vi "Swerve Out of loop.vi"(0 "x":dbl(slide)=-0.03937007874015748 scale=-1.0..1.0, 1 "Recalc offsets":bool, 2 "Recalc distance":bool, 5 "Rot. Point X":dbl, 7 "y":dbl(slide)=-0.07086614173228346 scale=-1.0..1.0, 9 "Rot. Point Y":dbl, 11 "z":dbl(knob)=-0.015748031496062992 scale=-1.0..1.0, 12 "Robot Centric":bool=TRUE, 13 "Auto Controls":bool) -> ()   [LabVIEW 2016]
uses:
  <vilib>/Rock Robotics/WPI/ThirdParty/CanMotor/TalonSRX/WPI_CANTalonSRX_APIControlMode.ctl
  <vilib>/Rock Robotics/WPI/ThirdParty/CanMotor/TalonSRX/WPI_CANTalonSRX_APIFeedbackSelect.ctl
  <vilib>/Rock Robotics/WPI/ThirdParty/CanMotor/TalonSRX/WPI_CANTalonSRX_StatusFrame.ctl
  <vilib>/Rock Robotics/Network Tables/NT Read Number.vi
  <vilib>/Rock Robotics/Network Tables/NT Read Numeric Array.vi
panel:
  in  "Default Offsets":dbl[](array[numeric])=[0.0987354, 0.084183, 0.097507, -0.49821]
  in  "negate feedback sensor":bool
  in  "Deadband":dbl=0.04 format="%#_13g"
  in  "Debug?":bool
  in  "Motor":bool[](array[boolean])=[FALSE, FALSE, FALSE, FALSE]
  in  "PIDF":cluster{"P":dbl, "I":dbl, "D":dbl, "F":dbl}={"P"=2.0, "I"=0.0, "D"=0.0, "F"=0.0}
  in  "Robot Width":dbl=26.0
  in  "Robot Length":dbl=22.125
  # "SWERVE DRIVE\nVersion 4.0\nCory Lynch\nChris Garuti\nGavin Popkin\nApple Pi Robotics\nTeam 2067"
  # "FL"
  # "FR"
  # "BL"
  # "BR"
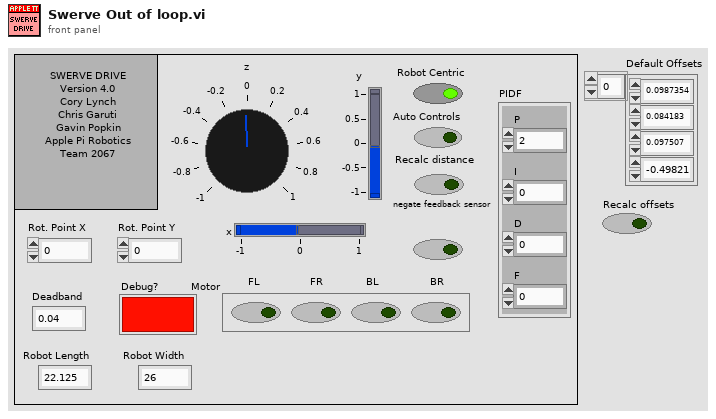
[diagram p1: front panel]
types:
  T1 = typedef "WPI_MotorControlDeviceRef.ctl" = cluster{"DeviceStatus":errorcluster, "Type":T2, "PWM":cluster{"PWM Channel":T3, "DeadBand":T4}, "CAN":cluster{"Device Number":u8, "SetOutput VI Ref":variant, "GetOutput VI Ref":variant, "Enable VI Ref":variant, "Disable VI Ref":variant, "Data":variant}, "Invert":bool}
  T2 = typedef "WPI_MotorControlType.ctl" = enum16{"PWM", "CAN"}
  T3 = typedef "FPGA_DIOPWMChannel.ctl" = enum8{"PWM 0", "PWM 1", "PWM 2", "PWM 3", "PWM 4", "PWM 5", "PWM 6", "PWM 7", "PWM 8", "PWM 9", "PWM MXP 0", "PWM MXP 1", "PWM MXP 2", "PWM MXP 3", "PWM MXP 4", "PWM MXP 5", "PWM MXP 6", "PWM MXP 7", "PWM MXP 8", "PWM MXP 9", "Invalid"}
  T4 = typedef "WPI_PWMDeadband.ctl" = cluster{"Name":string, "maxPositivePwm":i32, "minPositivePwm":i32, "centerPwm":i32, "maxNegativePwm":i32, "minNegativePwm":i32, "angularRange":u16}
  T5 = typedef "WPI_CANTalonSRX_StatusFrame.ctl" = enum16{"General Status Frame", "Feedback Status Frame", "Quadrature Status Frame", "Analog Temp Vbat Status Frame", "Pulse Width Status Frame"}
  T6 = typedef "WPI_CANTalonSRX_APIFeedbackSelect.ctl" = enum16{"Digital Quadrature Encoder", "Analog Potentiometer", "Analog Encoder", "Count on Quad-A (Rising-Edge)", "Count on Quad-A (Falling-Edge)", "CTR Magnetic Enc (Absolute)", "CTR Magnetic Enc (Relative)", "Pulse Width"}
  T7 = typedef "WPI_CANTalonSRX_GlobalStatus.ctl" = cluster{"Applied Throttle":dbl, "Module Enabled":bool, "CAN Error":errorcluster, "Closed Loop Error":dbl, "Forward Limit Switch Closed":bool, "Reverse Limit Switch Closed":bool, "Sensor Position":dbl, "Sensor Velocity":dbl, "Current":dbl, "Sticky Fault - Over Temp":bool, "Sticky Fault - Under Voltage":bool, "Sticky Fault - Forward Limit":bool, "Sticky Fault - Reverse Limit":bool, "Sticky Fault - Forward Soft Limit":bool, "Sticky Fault - Reverse Soft Limit":bool, "Brake is Enabled":bool, "Encoder Position":dbl, "Encoder Velocity":dbl, "Encoder Index Count":dbl, "Encoder A Pin State":bool, "Encoder B Pin State":bool, "Encoder Index Pin State":bool, "Analog In":dbl, "Analog In Velocity":dbl, "Temperature (C)":dbl, "Battery Voltage":dbl, "Control 5 Is Supported":bool, "Current Profile Slot Select":dbl, "Pos Div 8":bool, "Vel Div 4":bool, "Pulse Width Position":i32, "Pulse Width Velocity":i32, "Pulse Width Rise To Rise (us)":i32, "Pulse Width Rise To Fall (us)":i32, "Mot Prof Active Is Under Run":bool, "Mot Prof Active Has Under Run":bool, "Mot Prof Active Is Last":bool, "Mot Prof Active Velocity Only":bool, "Mot Prof Active Is Valid":bool, "Mot Prof Buffer Is Full":bool, "Mot Prof Active Profile Slot Select":i32, "Mot Prof NextID":i32, "Mot Prof Count":i32, "Mot Prof Active Velocity":dbl, "Mot Prof Active Position":dbl, "Mot Prof Output Enable":i32, "UsageFrame":u32, "Motion Magic Active Trajectory":cluster{"Velocity":dbl, "Position":dbl}}
  T8 = typedef "WPI_CANTalonSRX_APIControlMode.ctl" = enum8{"Percent VBus", "Speed", "Position", "Slave", "Unchanged / Invalid", "Voltage Compensation", "Current", "Motion Profile", "Motion Magic"}
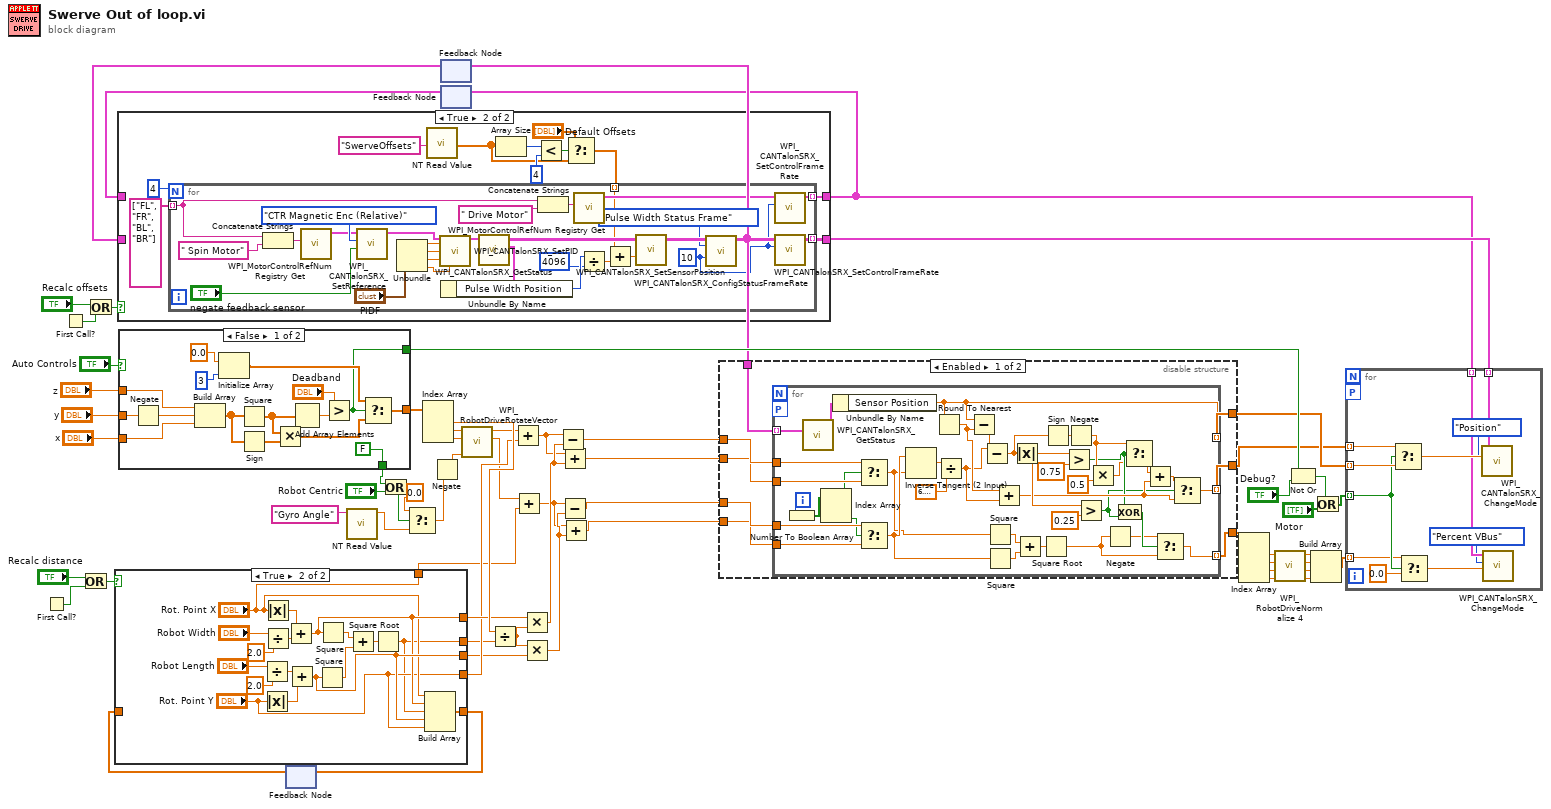
[diagram p0: block diagram]
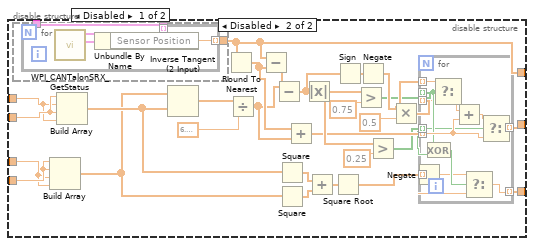
[diagram p2: hidden frame]
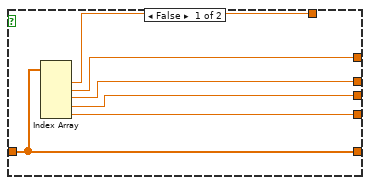
[diagram p5: hidden frame]
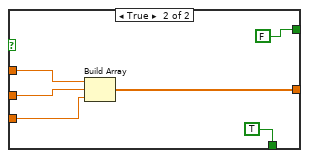
[diagram p6: hidden frame]
diagram:
  n1 = First Call?() -> (First Call?: T/F=w38:bool)
  n2 = First Call?() -> (First Call?: T/F=w12:bool)
  n3 = Or(x="Recalc distance", y=w38) -> (x .or. y?=w36:bool)
  n4 = Or(x="Recalc offsets", y=w12) -> (x .or. y?=w39:bool)
  n5 = case shown="False" "Auto Controls" {
    tunnel: [w71 w83] -> w61
    tunnel: [w67 FALSE] -> w51
    tunnel: "z" -> [w65 w81]
    tunnel: "y" -> [w64 w80]
    tunnel: "x" -> [w63 w79]
    tunnel: [FALSE TRUE] -> w3
    frame False {
      n6 = Negate(x=w64) -> (-x=w66:dbl)
      n7 = Build Array(w65, w66, w63) -> (w75:dbl[])
      n8 = Initialize Array(0.0 ("element"), 3 ("dimension size")) -> (w77:dbl[])
      n9 = Square(x=w75) -> (x^2=w73:dbl[])
      n10 = Sign(1:w75) -> (0:w74:dbl[])
      n11 = Multiply(x=w73, y=w74) -> (x*y=w72:dbl[])
      n12 = Add Array Elements(numeric array=w73) -> (sum=w69:dbl)
      n13 = Greater?(x="Deadband", y=w69) -> (0:w67:bool)
      n14 = Select(t=w77, s=w67, f=w72) -> (s? t:f=w71:dbl[])
    }
    frame True {
      n15 = Build Array(w81, w80, w79) -> (w83:dbl[])
    }
  }
  n16 = feedback #1() -> (w20:dbl[])  [unwired: 1 in]
  n17 = case shown="True" w36 {
    tunnel: [w88 w94] -> w58
    tunnel: [w85 "Rot. Point Y"] -> w57
    tunnel: [w89 "Rot. Point X"] -> w30
    tunnel: [w87 w90] -> w55
    tunnel: [w86 w95] -> w56
    tunnel: [w84 w91] -> w19
    tunnel: w20 -> [w84 _]
    frame False {
      n18 = Index Array(array=w84) -> (element #1=w89:dbl, element #2=w88:dbl, element #3=w87:dbl, element #4=w86:dbl, element #5=w85:dbl)  [unwired: 5 in]
    }
    frame True {
      n19 = Divide(x="Robot Length", y=2.0) -> (x/y=w98:dbl)
      n20 = Absolute Value(x="Rot. Point Y") -> (abs(x)=w97:dbl)
      n21 = Absolute Value(x="Rot. Point X") -> (abs(x)=w96:dbl)
      n22 = Divide(x="Robot Width", y=2.0) -> (x/y=w99:dbl)
      n23 = Add(x=w96, y=w99) -> (x+y=w94:dbl)
      n24 = Add(x=w98, y=w97) -> (x+y=w95:dbl)
      n25 = Square(x=w95) -> (x^2=w101:dbl)
      n26 = Square(x=w94) -> (x^2=w104:dbl)
      n27 = Add(x=w104, y=w101) -> (x+y=w105:dbl)
      n28 = Square Root(x=w105) -> (sqrt(x)=w90:dbl)
      n29 = Build Array("Rot. Point X", w94, w90, w95, "Rot. Point Y") -> (w91:dbl[])
    }
  }
  n30 = feedback-in #1(w19) -> ()
  n31 = call-poly <vilib>:"NT Read Value.vi"("Name"="Gyro Angle") -> ("Numeric"=w1:dbl)  [unwired: 9 in, 1 out]
  n32 = Or(x=w3, y="Robot Centric") -> (x .or. y?=w4:bool)
  n33 = Select(t=0.0, s=w4, f=w1) -> (s? t:f=w49:dbl)
  n34 = Index Array(array=w61) -> (element #1=w60:dbl, element #2=w48:dbl, element #3=w47:dbl)  [unwired: 3 in]
  n35 = Negate(x=w49) -> (-x=w11:dbl)
  n36 = feedback #2() -> (w16:T1[])  [unwired: 1 in]
  n37 = feedback #3() -> (w18:T1[])  [unwired: 1 in]
  n38 = case shown="True" w39 {
    tunnel: [w107 w119] -> w17
    tunnel: [w108 w118] -> w15
    tunnel: w18 -> [w108 _]
    tunnel: w16 -> [w107 _]
    frame False {
    }
    frame True {
      n39 = call-poly <vilib>:"NT Read Value.vi"("Name"="SwerveOffsets") -> ("Numeric Array"=w110:dbl[])  [unwired: 9 in, 1 out]
      n40 = Array Size(array=w110) -> (size(s)=w115:i32)
      n41 = Less?(x=w115, y=4) -> (x < y?=w113:bool)
      n42 = Select(t="Default Offsets", s=w113, f=w110) -> (s? t:f=w111:dbl[])
      n43 = for {
        N: 4 -> [_]
        tunnel: string[] ["FL", "FR", "BL", "BR"] -> [w142] mode=indexing
        tunnel: [w121] -> w118 mode=indexing
        tunnel: [w122] -> w119 mode=indexing
        tunnel: w111 -> [w125] mode=indexing
        w120 = u32 10 ("Frame Rate Ms")
        n44 = Concatenate Strings(w142, " Spin Motor" ("refnum name")) -> (w141:string)
        n45 = call <vilib>:"WPI_MotorControlRefNum Registry Get.vi"("refnum name"=w141) -> ("MotorControlDevRef"=w143:T1)  [unwired: 9 in, 1 out]
        n46 = call <vilib>:"WPI_CANTalonSRX_SetReference.vi"("Reverse Feedback Sensor"="negate feedback sensor", "Feedback Reference"=WPI_CANTalonSRX_APIFeedbackSelect."CTR Magnetic Enc (Relative)", "CAN Talon SRX Ref"=w143) -> ("CAN Talon SRX Ref"=w137:T1)  [unwired: 7 in, 1 out]
        n47 = Unbundle("PIDF") -> ("P"=w144:dbl, "I"=w146:dbl, "D"=w145:dbl, "F"=w135:dbl)
        n48 = call <vilib>:"WPI_CANTalonSRX_SetPID.vi"("CAN Talon SRX Ref"=w137, "P"=w144, "I"=w146, "D"=w145, "F"=w135) -> ("CAN Talon SRX Ref"=w133:T1)  [unwired: 9 in, 1 out]
        n49 = call <vilib>:"WPI_CANTalonSRX_GetStatus.vi"("CAN Talon SRX Ref"=w133) -> ("Talon SRX Status"=w130:T7, "CAN Talon SRX Ref"=w132:T1)  [unwired: 8 in, 1 out]
        n50 = Unbundle By Name(w130) -> ("Pulse Width Position"=w128:i32)
        n51 = Concatenate Strings(w142, " Drive Motor") -> (w140:string)
        n52 = call <vilib>:"WPI_MotorControlRefNum Registry Get.vi"("refnum name"=w140) -> ("MotorControlDevRef"=w139:T1)  [unwired: 9 in, 1 out]
        n53 = Divide(x=w128, y=4096) -> (x/y=w129:dbl)
        n54 = Add(x=w125, y=w129) -> (x+y=w126:dbl)
        n55 = call <vilib>:"WPI_CANTalonSRX_SetSensorPosition.vi"("New Sensor Position"=w126, "CAN Talon SRX Ref"=w132) -> ("CAN Talon SRX Ref"=w131:T1)  [unwired: 8 in, 1 out]
        n56 = call <vilib>:"WPI_CANTalonSRX_ConfigStatusFrameRate.vi"("CAN Talon SRX Ref"=w131, "Talon SRX Status Frame"=WPI_CANTalonSRX_StatusFrame."Pulse Width Status Frame", "Frame Rate Ms"=w120) -> ("CAN Talon SRX Ref"=w124:T1)  [unwired: 12 in]
        n57 = call <vilib>:"WPI_CANTalonSRX_SetControlFrameRate.vi"("Control Frame Rate (ms)"=w120, "CAN Talon SRX Ref"=w139) -> ("CAN Talon SRX Ref"=w121:T1)  [unwired: 8 in, 1 out]
        n58 = call <vilib>:"WPI_CANTalonSRX_SetControlFrameRate.vi"("Control Frame Rate (ms)"=w120, "CAN Talon SRX Ref"=w124) -> ("CAN Talon SRX Ref"=w122:T1)  [unwired: 8 in, 1 out]
      }
    }
  }
  n59 = feedback-in #2(w17) -> ()
  n60 = feedback-in #3(w15) -> ()
  n61 = call <vilib>:"WPI_RobotDriveRotateVector.vi"("Angle"=w11, "X"=w47, "Y"=w48) -> ("X'"=w45:dbl, "Y'"=w46:dbl)  [unwired: 7 out]
  n62 = Divide(x=w60, y=w55) -> (x/y=w59:dbl)
  n63 = Add(x=w46, y=w57) -> (x+y=w31:dbl)
  n64 = Add(x=w45, y=w30) -> (x+y=w32:dbl)
  n65 = Multiply(x=w58, y=w59) -> (x*y=w34:dbl)
  n66 = Multiply(x=w59, y=w56) -> (x*y=w33:dbl)
  n67 = Subtract(x=w31, y=w34) -> (x-y=w10:dbl)
  n68 = Add(x=w31, y=w34) -> (x+y=w9:dbl)
  n69 = Subtract(x=w32, y=w33) -> (x-y=w8:dbl)
  n70 = Add(x=w32, y=w33) -> (x+y=w7:dbl)
  n71 = disable-structure shown="Enabled" {
    disable-tunnel: [w156 w197] -> w35
    disable-tunnel: [w155 w198] -> w29
    disable-tunnel: [w154 w200] -> w24
    disable-tunnel: w17 -> [w153 w199]
    disable-tunnel: w10 -> [w152 w205]
    disable-tunnel: w9 -> [w151 w206]
    disable-tunnel: w8 -> [w150 w202]
    disable-tunnel: w7 -> [w149 w203]
    frame Enabled {
      n72 = for {
        tunnel: [w191] -> w155 mode=indexing
        tunnel: [w168] -> w154 mode=indexing
        tunnel: w153 -> [w188] mode=indexing
        tunnel: [w175] -> w156 mode=indexing
        tunnel: w152 -> [w182]
        tunnel: w151 -> [w183]
        tunnel: w150 -> [w185]
        tunnel: w149 -> [w184]
        workers-P: _ -> [_]
        i -> [w187]
        n73 = Number To Boolean Array(number=w187) -> (Boolean array=w186:bool[])
        n74 = call <vilib>:"WPI_CANTalonSRX_GetStatus.vi"("CAN Talon SRX Ref"=w188) -> ("Talon SRX Status"=w157:T7)  [unwired: 8 in, 2 out]
        n75 = Index Array(array=w186) -> (element #1=w159:bool, element #2=w158:bool)  [unwired: 2 in]
        n76 = Unbundle By Name(w157) -> ("Sensor Position"=w175:dbl)
        n77 = Select(t=w182, s=w159, f=w183) -> (s? t:f=w180:dbl)
        n78 = Select(t=w185, s=w158, f=w184) -> (s? t:f=w181:dbl)
        n79 = Inverse Tangent (2 Input)(1:w180, 2:w181) -> (0:w189:dbl)
        n80 = Round To Nearest(number=w175) -> (nearest integer value=w173:dbl)
        n81 = Divide(x=w189, y=6.283185307179586) -> (x/y=w172:dbl)
        n82 = Subtract(x=w175, y=w173) -> (x-y=w179:dbl)
        n83 = Subtract(x=w172, y=w179) -> (x-y=w174:dbl)
        n84 = Square(x=w180) -> (x^2=w194:dbl)
        n85 = Square(x=w181) -> (x^2=w195:dbl)
        n86 = Add(x=w173, y=w172) -> (x+y=w167:dbl)
        n87 = Absolute Value(x=w174) -> (abs(x)=w177:dbl)
        n88 = Add(x=w194, y=w195) -> (x+y=w193:dbl)
        n89 = Square Root(x=w193) -> (sqrt(x)=w192:dbl)
        n90 = Sign(1:w174) -> (0:w170:dbl)
        n91 = Greater?(x=w177, y=0.75) -> (0:w165:bool)
        n92 = Negate(x=w170) -> (-x=w166:dbl)
        n93 = Greater?(x=w177, y=0.25) -> (0:w160:bool)
        n94 = Multiply(x=w166, y=0.5) -> (x*y=w163:dbl)
        n95 = Negate(x=w192) -> (-x=w161:dbl)
        n96 = Exclusive Or(1:w160, 2:w165) -> (0:w164:bool)
        n97 = Select(t=w166, s=w165, f=w163) -> (s? t:f=w169:dbl)
        n98 = Add(x=w169, y=w167) -> (x+y=w162:dbl)
        n99 = Select(t=w161, s=w164, f=w192) -> (s? t:f=w191:dbl)
        n100 = Select(t=w162, s=w160, f=w167) -> (s? t:f=w168:dbl)
      }
    }
    frame Disabled {
      n101 = disable-structure shown="Disabled" {
        disable-tunnel: w199 -> [w227 _]
        disable-tunnel: [w226 _] -> w197
        frame Disabled {
          n102 = for {
            tunnel: [w228] -> w226 mode=indexing
            tunnel: w227 -> [w230] mode=indexing
            n103 = call <vilib>:"WPI_CANTalonSRX_GetStatus.vi"("CAN Talon SRX Ref"=w230) -> ("Talon SRX Status"=w229:T7)  [unwired: 8 in, 2 out]
            n104 = Unbundle By Name(w229) -> ("Sensor Position"=w228:dbl)
          }
        }
        frame Enabled {
        }
      }
      n105 = Build Array(w203, w203, w202, w202) -> (w201:dbl[])
      n106 = Build Array(w206, w205, w206, w205) -> (w204:dbl[])
      n107 = Inverse Tangent (2 Input)(1:w204, 2:w201) -> (0:w220:dbl[])
      n108 = Round To Nearest(number=w197) -> (nearest integer value=w214:dbl[])
      n109 = Divide(x=w220, y=6.283185307179586) -> (x/y=w213:dbl[])
      n110 = Subtract(x=w197, y=w214) -> (x-y=w219:dbl[])
      n111 = Subtract(x=w213, y=w219) -> (x-y=w215:dbl[])
      n112 = Square(x=w204) -> (x^2=w224:dbl[])
      n113 = Square(x=w201) -> (x^2=w225:dbl[])
      n114 = Add(x=w214, y=w213) -> (x+y=w210:dbl[])
      n115 = Absolute Value(x=w215) -> (abs(x)=w217:dbl[])
      n116 = Add(x=w224, y=w225) -> (x+y=w223:dbl[])
      n117 = Square Root(x=w223) -> (sqrt(x)=w222:dbl[])
      n118 = Sign(1:w215) -> (0:w211:dbl[])
      n119 = Greater?(x=w217, y=0.75) -> (0:w208:bool[])
      n120 = Negate(x=w211) -> (-x=w209:dbl[])
      n121 = Greater?(x=w217, y=0.25) -> (0:w207:bool[])
      n122 = Multiply(x=w209, y=0.5) -> (x*y=w196:dbl[])
      n123 = for {
        tunnel: w222 -> [w242] mode=indexing
        tunnel: w210 -> [w240] mode=indexing
        tunnel: w209 -> [w239] mode=indexing
        tunnel: w208 -> [w238] mode=indexing
        tunnel: w196 -> [w236] mode=indexing
        tunnel: w207 -> [w233] mode=indexing
        tunnel: [w232] -> w200 mode=indexing
        tunnel: [w231] -> w198 mode=indexing
        n124 = Negate(x=w242) -> (-x=w234:dbl)
        n125 = Exclusive Or(1:w233, 2:w238) -> (0:w237:bool)
        n126 = Select(t=w239, s=w238, f=w236) -> (s? t:f=w241:dbl)
        n127 = Add(x=w241, y=w240) -> (x+y=w235:dbl)
        n128 = Select(t=w234, s=w237, f=w242) -> (s? t:f=w231:dbl)
        n129 = Select(t=w235, s=w233, f=w240) -> (s? t:f=w232:dbl)
      }
    }
  }
  n130 = Index Array(array=w29) -> (element #1=w28:dbl, element #2=w27:dbl, element #3=w26:dbl, element #4=w25:dbl)  [unwired: 4 in]
  n131 = call <vilib>:"WPI_RobotDriveNormalize 4.vi"("D"=w25, "C"=w26, "B"=w27, "A"=w28) -> ("D'"=w43:dbl, "C'"=w42:dbl, "B'"=w41:dbl, "A'"=w44:dbl)
  n132 = Not Or(1:"Debug?", 2:w51) -> (0:w50:bool)
  n133 = Build Array(w44, w41, w42, w43) -> (w40:dbl[])
  n134 = Or(x=w50, y="Motor") -> (x .or. y?=w54:bool[])
  n135 = for {
    tunnel: w24 -> [w248] mode=indexing
    tunnel: w17 -> [w253] mode=indexing
    tunnel: w54 -> [w247] mode=indexing
    tunnel: w35 -> [w250] mode=indexing
    tunnel: w40 -> [w246] mode=indexing
    tunnel: w15 -> [w245] mode=indexing
    workers-P: _ -> [_]
    n136 = Select(t=w248, s=w247, f=w250) -> (s? t:f=w249:dbl)
    n137 = Select(t=w246, s=w247, f=0.0) -> (s? t:f=w252:dbl)
    n138 = call <vilib>:"WPI_CANTalonSRX_ChangeMode.vi"("Output"=w249, "Control Mode"=WPI_CANTalonSRX_APIControlMode."Position", "CAN Talon SRX Ref"=w253) -> ()  [unwired: 7 in, 2 out]
    n139 = call <vilib>:"WPI_CANTalonSRX_ChangeMode.vi"("Output"=w252, "Control Mode"=WPI_CANTalonSRX_APIControlMode."Percent VBus", "CAN Talon SRX Ref"=w245) -> ()  [unwired: 7 in, 2 out]
  }
